vi "Y_Limiter Run.vi"(5 "reinitialize? (F)":bool, 7 "X1(SetState)":T1(ring)=enum."max", 9 "Y (NaN)":dbl=nan, 10 "Y_Set":dbl, 11 "Y_Limiter in":refnum<class "Y_Limiter.lvclass">) -> (1 "output":dbl format="%.2f", 2 "Y_Lim_State":T2=enum."increase", 3 "Y_Limiter out":refnum<class "Y_Limiter.lvclass">, 4 "End":bool)   [LabVIEW 2019, in "control.lvlib" / "Y_Limiter.lvclass"]
uses:
  Y_Limiter.lvclass
  ctl/Y_Lim_State.ctl
  control.lvlib
  PID/PID Output Rate Limiter/PID Output Rate Limiter.lvclass
  D:/my_projects/projects/Algorithms/Labview/19/Reg/PID/PID Output Rate Limiter/PID Output Rate Limiter.lvclass
  D:/my_projects/projects/Algorithms/Labview/19/Reg/PID/PID Timing Estimation/PID Timing Estimation.lvclass
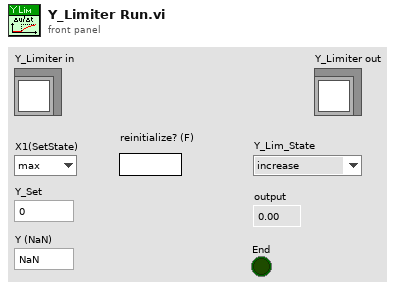
[diagram p1: front panel]
types:
  T1 = enum8{"alarm", "min", "stop", "hand", "auto", "max"}
  T2 = typedef "control.lvlib/Y_Lim_State.ctl" = enum8{"initialization", "alarm", "stop", "decrease", "increase"}
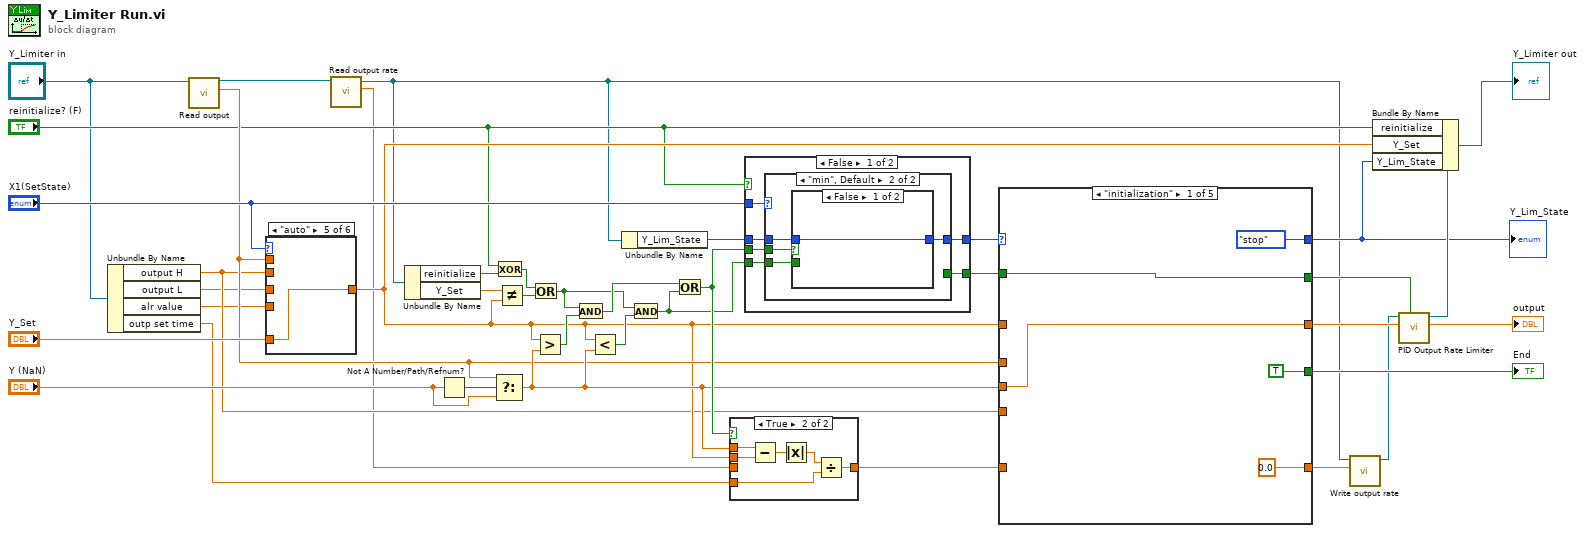
[diagram p0: block diagram]
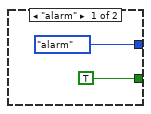
[diagram p7: hidden frame]
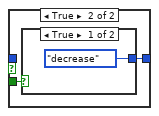
[diagram p8: hidden frame]
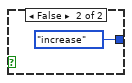
[diagram p9: hidden frame]
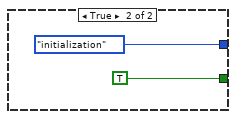
[diagram p10: hidden frame]
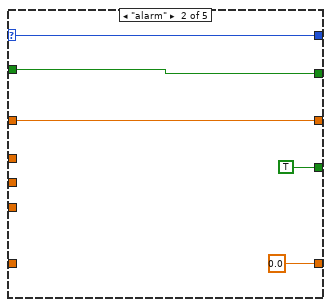
[diagram p12: hidden frame]
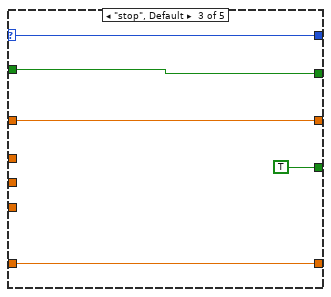
[diagram p13: hidden frame]
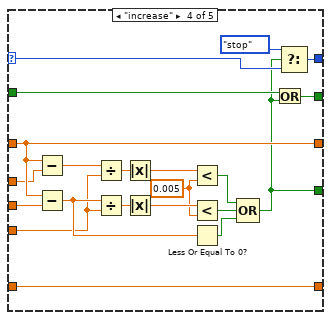
[diagram p14: hidden frame]
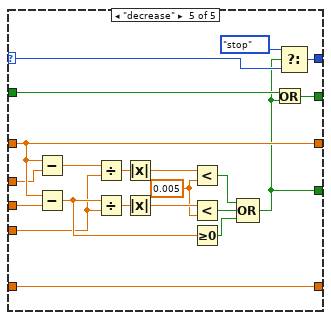
[diagram p15: hidden frame]
diagram:
  n1 = Unbundle By Name("Y_Limiter in") -> ("output H"=w8:dbl, "output L"=w7:dbl, "alr value"=w6:dbl, "outp set time"=w5:dbl)
  n2 = call "Read output.vi"("PID Output Rate Limiter in"="Y_Limiter in") -> ("output"=w19:dbl, "PID Output Rate Limiter out"=w2:refnum<class "Y_Limiter.lvclass">)  [unwired: 9 in]
  n3 = case shown="\"auto\"" "X1(SetState)" {
    tunnel: w8 -> [_ _ _ _ _ w45]
    tunnel: w6 -> [w40 _ _ _ _ _]
    tunnel: w7 -> [_ w41 _ _ _ _]
    tunnel: "Y_Set" -> [_ _ _ w43 w44 _]
    tunnel: [w40 w41 w42 w43 w44 w45] -> w12
    tunnel: w19 -> [_ _ w42 _ _ _]
    frame "alarm", Default {
    }
    frame "min" {
    }
    frame "stop" {
    }
    frame "hand" {
    }
    frame "auto" {
    }
    frame "max" {
    }
  }
  n4 = call "Read output rate.vi"("PID Output Rate Limiter in"=w2) -> ("output rate"=w4:dbl, "PID Output Rate Limiter out"=w1:refnum<class "Y_Limiter.lvclass">)  [unwired: 9 in]
  n5 = Unbundle By Name(w1) -> ("reinitialize"=w13:bool, "Y_Set"=w15:dbl)
  n6 = Not A Number/Path/Refnum?(number/path/refnum="Y (NaN)") -> (NaN/Path/Refnum?=w34:bool)
  n7 = Select(t=w19, s=w34, f="Y (NaN)") -> (s? t:f=w21:dbl)
  n8 = Exclusive Or(1:w13, 2:"reinitialize? (F)") -> (0:w22:bool)
  n9 = Not Equal?(x=w15, y=w12) -> (x != y?=w30:bool)
  n10 = Or(x=w22, y=w30) -> (x .or. y?=w23:bool)
  n11 = Greater?(x=w12, y=w21) -> (0:w32:bool)
  n12 = And(x=w23, y=w32) -> (x .and. y?=w31:bool)
  n13 = Less?(x=w12, y=w21) -> (x < y?=w29:bool)
  n14 = Unbundle By Name(w1) -> ("Y_Lim_State"=w14:T2)
  n15 = And(x=w23, y=w29) -> (x .and. y?=w9:bool)
  n16 = Or(x=w31, y=w9) -> (x .or. y?=w27:bool)
  n17 = case shown="True" w27 {
    tunnel: w21 -> [_ w47]
    tunnel: w12 -> [_ w48]
    tunnel: w4 -> [w46 _]
    tunnel: [w46 w50] -> w35
    tunnel: w5 -> [_ w49]
    frame False {
    }
    frame True {
      n18 = Subtract(x=w47, y=w48) -> (x-y=w51:dbl)
      n19 = Absolute Value(x=w51) -> (abs(x)=w52:dbl)
      n20 = Divide(x=w52, y=w49) -> (x/y=w50:dbl)
    }
  }
  n21 = case shown="False" "reinitialize? (F)" {
    tunnel: [w57 Y_Lim_State."initialization" ("SpLim_State")] -> w26
    tunnel: [w53 TRUE] -> w24
    tunnel: w27 -> [w58 _]
    tunnel: w9 -> [w56 _]
    tunnel: w14 -> [w55 _]
    tunnel: "X1(SetState)" -> [w54 _]
    frame False {
      n22 = case shown="\"min\", Default" w54 {
        tunnel: w58 -> [_ w64]
        tunnel: [Y_Lim_State."alarm" ("SpLim_State") w63] -> w57
        tunnel: w56 -> [_ w62]
        tunnel: w55 -> [_ w61]
        tunnel: [TRUE _] -> w53
        frame "alarm" {
        }
        frame "min", Default {
          n23 = case shown="False" w64 {
            tunnel: [w65 w67] -> w63
            tunnel: w62 -> [_ w66]
            tunnel: w61 -> [w65 _]
            frame False {
            }
            frame True {
              n24 = case shown="True" w66 {
                tunnel: [Y_Lim_State."decrease" ("SpLim_State") Y_Lim_State."increase" ("SpLim_State")] -> w67
                frame True {
                }
                frame False {
                }
              }
            }
          }
        }
      }
    }
    frame True {
    }
  }
  n25 = case shown="\"initialization\"" w26 {
    selector: w26 -> [_ w77 w84 w100 w121]
    tunnel: w12 -> [_ w78 w85 w98 w119]
    tunnel: w21 -> [w74 _ _ w93 w114]
    tunnel: [w74 w78 w85 w98 w119] -> w36
    tunnel: [TRUE TRUE TRUE w87 w108] -> w38
    tunnel: [0.0 0.0 w83 w103 w124] -> w18
    tunnel: [w73 w79 w82 w88 w110] -> w37
    tunnel: [Y_Lim_State."stop" ("t") w77 w84 w101 w122] -> w11
    tunnel: w35 -> [_ _ w83 w103 w124]
    tunnel: w19 -> [_ _ _ w97 w118]
    tunnel: w8 -> [_ _ _ w91 w112]
    tunnel: w24 -> [w73 w79 w82 w89 w109]
    frame "initialization" {
    }
    frame "alarm" {
    }
    frame "stop", Default {
    }
    frame "increase" {
      w90 = 0.005 ("y")
      n26 = Subtract(x=w98, y=w97) -> (x-y=w94:dbl)
      n27 = Subtract(x=w98, y=w93) -> (x-y=w102:dbl)
      n28 = Divide(x=w94, y=w91) -> (x/y=w95:dbl)
      n29 = Divide(x=w102, y=w91) -> (x/y=w107:dbl)
      n30 = Absolute Value(x=w95) -> (abs(x)=w96:dbl)
      n31 = Absolute Value(x=w107) -> (abs(x)=w106:dbl)
      n32 = Less?(x=w96, y=w90) -> (x < y?=w92:bool)
      n33 = Less?(x=w106, y=w90) -> (x < y?=w105:bool)
      n34 = Less Or Equal To 0?(x=w102) -> (x <= 0?=w104:bool)
      n35 = Compound Arithmetic op=OR(w92, w105, w104) -> (w87:bool)
      n36 = Or(x=w89, y=w87) -> (x .or. y?=w88:bool)
      n37 = Select(t=Y_Lim_State."stop", s=w87, f=w100) -> (s? t:f=w101:T2)
    }
    frame "decrease" {
      w111 = 0.005 ("y")
      n38 = Subtract(x=w119, y=w118) -> (x-y=w115:dbl)
      n39 = Subtract(x=w119, y=w114) -> (x-y=w123:dbl)
      n40 = Divide(x=w115, y=w112) -> (x/y=w116:dbl)
      n41 = Divide(x=w123, y=w112) -> (x/y=w128:dbl)
      n42 = Absolute Value(x=w116) -> (abs(x)=w117:dbl)
      n43 = Absolute Value(x=w128) -> (abs(x)=w127:dbl)
      n44 = Less?(x=w117, y=w111) -> (x < y?=w113:bool)
      n45 = Less?(x=w127, y=w111) -> (x < y?=w126:bool)
      n46 = Greater Or Equal To 0?(x=w123) -> (x >= 0?=w125:bool)
      n47 = Compound Arithmetic op=OR(w113, w126, w125) -> (w108:bool)
      n48 = Or(x=w109, y=w108) -> (x .or. y?=w110:bool)
      n49 = Select(t=Y_Lim_State."stop", s=w108, f=w121) -> (s? t:f=w122:T2)
    }
  }
  "End" <- w38
  "Y_Lim_State" <- w11
  n50 = call "Write output rate.vi"("output rate"=w18, "PID Output Rate Limiter in"=w1) -> ("PID Output Rate Limiter out"=w16:refnum<class "Y_Limiter.lvclass">)  [unwired: 9 in]
  n51 = call "PID Output Rate Limiter.vi"("reinitialize? (F)"=w37, "input (controller output)"=w36, "PID Output Rate Limiter in"=w16) -> ("output"=→"output":dbl, "PID Output Rate Limiter out"=w17:refnum<class "Y_Limiter.lvclass">)  [unwired: 6 in, 1 out]
  n52 = Bundle By Name(cluster=w17, "reinitialize"="reinitialize? (F)", "Y_Set"=w12, "Y_Lim_State"=w11) -> (→"Y_Limiter out":refnum<class "Y_Limiter.lvclass">)
